vi "PMOD Example(FPGA).vi"() -> ()   [LabVIEW 2013]
uses:
  <vilib>/rvi/DataTransferAndStorage/Container/XNode/niFpgaContainer.xnode
  <vilib>/rvi/interface/RandomDataEmulation/nirviRandomDataFpgaReadWriteTemplate.vi
  <vilib>/Platform/TimedLoop/XDataNode/XDataNode.xnode
  <vilib>/Platform/TimedLoop/XDataNode/nitl_modes.ctl
  <vilib>/Platform/TimedLoop/XDataNode/XDNodeRunTimeDep.lvlib
  <vilib>/Platform/TimedLoop/XDataNode/wakeup.ctl
  <vilib>/Platform/TimedLoop/XDataNode/timing_clust.ctl
  DIO/SPI Digital IO Lines.ctl
  DIO/SPI DIO Enable Lines.ctl
  Controls/SPIExample.CurrentStateFPGA.ctl
  <userlib>/_NI SPI IP/FPGA/Controllers/Public/Spi Master Outputs.ctl
  <userlib>/_NI SPI IP/FPGA/Controllers/NI SPI IP (FPGA).lvlib
  <userlib>/_NI SPI IP/FPGA/Controllers/Public/Transfer Settings.ctl
panel:
  out "Raw ADC Data":u64
  out "read Iterations":i32
  in  "Data To ADC":u64=2147483648
  in  "Chip Select":u8
  in  "SPI PHY Settings":T1={"Divide Value"=20, "Transfer Length (bits)"=32, "CS Asserted Polarity"=FALSE, "Clock Polarity (CPOL)"=FALSE, "Clock Phase (CPHA)"=FALSE, "Lengthen MISO Setup"=FALSE, "Direction Change Bit"=0, "MOSI Starts as Output"=FALSE, "Tristatable MOSI"=FALSE} {"Direction Change Bit" max=64 step=1; "Transfer Length (bits)" min=1 max=64 step=1}
  out "spi output":T2
  in  "Chan Offset Array":sgl[](array[numeric])=[0.0, 0.0, 0.0, 0.0, 0.0, 0.0, 0.0, 0.0, 0.0, 0.0, 0.0, 0.0, 0.0, 0.0, 0.0, 0.0, 0.0, 0.0, 0.0, 0.0, 0.0, 0.0, 0.0, 0.0, 0.0, 0.0, 0.0, 0.0, 0.0, 0.0, 0.0, 0.0, 0.0, 0.0, 0.0, 0.0, 0.0, 0.0, 0.0, 0.0]
  out "SGL Data":sgl
  out "State":T3
  out "Iterations":i32
  in  "Debug":bool=TRUE
  out "Chan Count":bool
  out "oclk mult":u32
  in  "data rate (S/s)":u32=10000
  out "oclk freq":u32
  out "oclk div":u32
  in  "Chan Scale Array":sgl[](array[numeric])=[1.0, 1.0, 1.0, 0.0, 0.0, 0.0, 0.0, 0.0, 0.0, 0.0, 0.0, 0.0, 0.0, 0.0, 0.0, 0.0, 0.0, 0.0, 0.0, 0.0, 0.0, 0.0, 0.0, 0.0, 0.0, 0.0, 0.0, 0.0, 0.0, 0.0, 0.0, 0.0, 0.0, 0.0, 0.0, 0.0, 0.0, 0.0, 0.0, 0.0]
  out "FPGA Error":errorcluster
  out "Finished":bool
  in  "stop":bool
  out "Module Underflow":bool
  out "Acq Loop Ticks":u32
  out "DMA FIFO Full":bool
  out "First Read":bool
  in  "Number of Channels":i32=4
  in  "Acquisition Type":enum16{"Finite Samples", "Continuous Samples"}(ring)=enum."Continuous Samples"
  in  "Samps per Chan [Finite]":i32=5120
  # "OUTPUT"
  # "INPUT"
  # "ADC Data::Debug"
  # "Acquisition Parameters"
  # "SPI PHY Settings"
  # "Debug"
  # "Status"
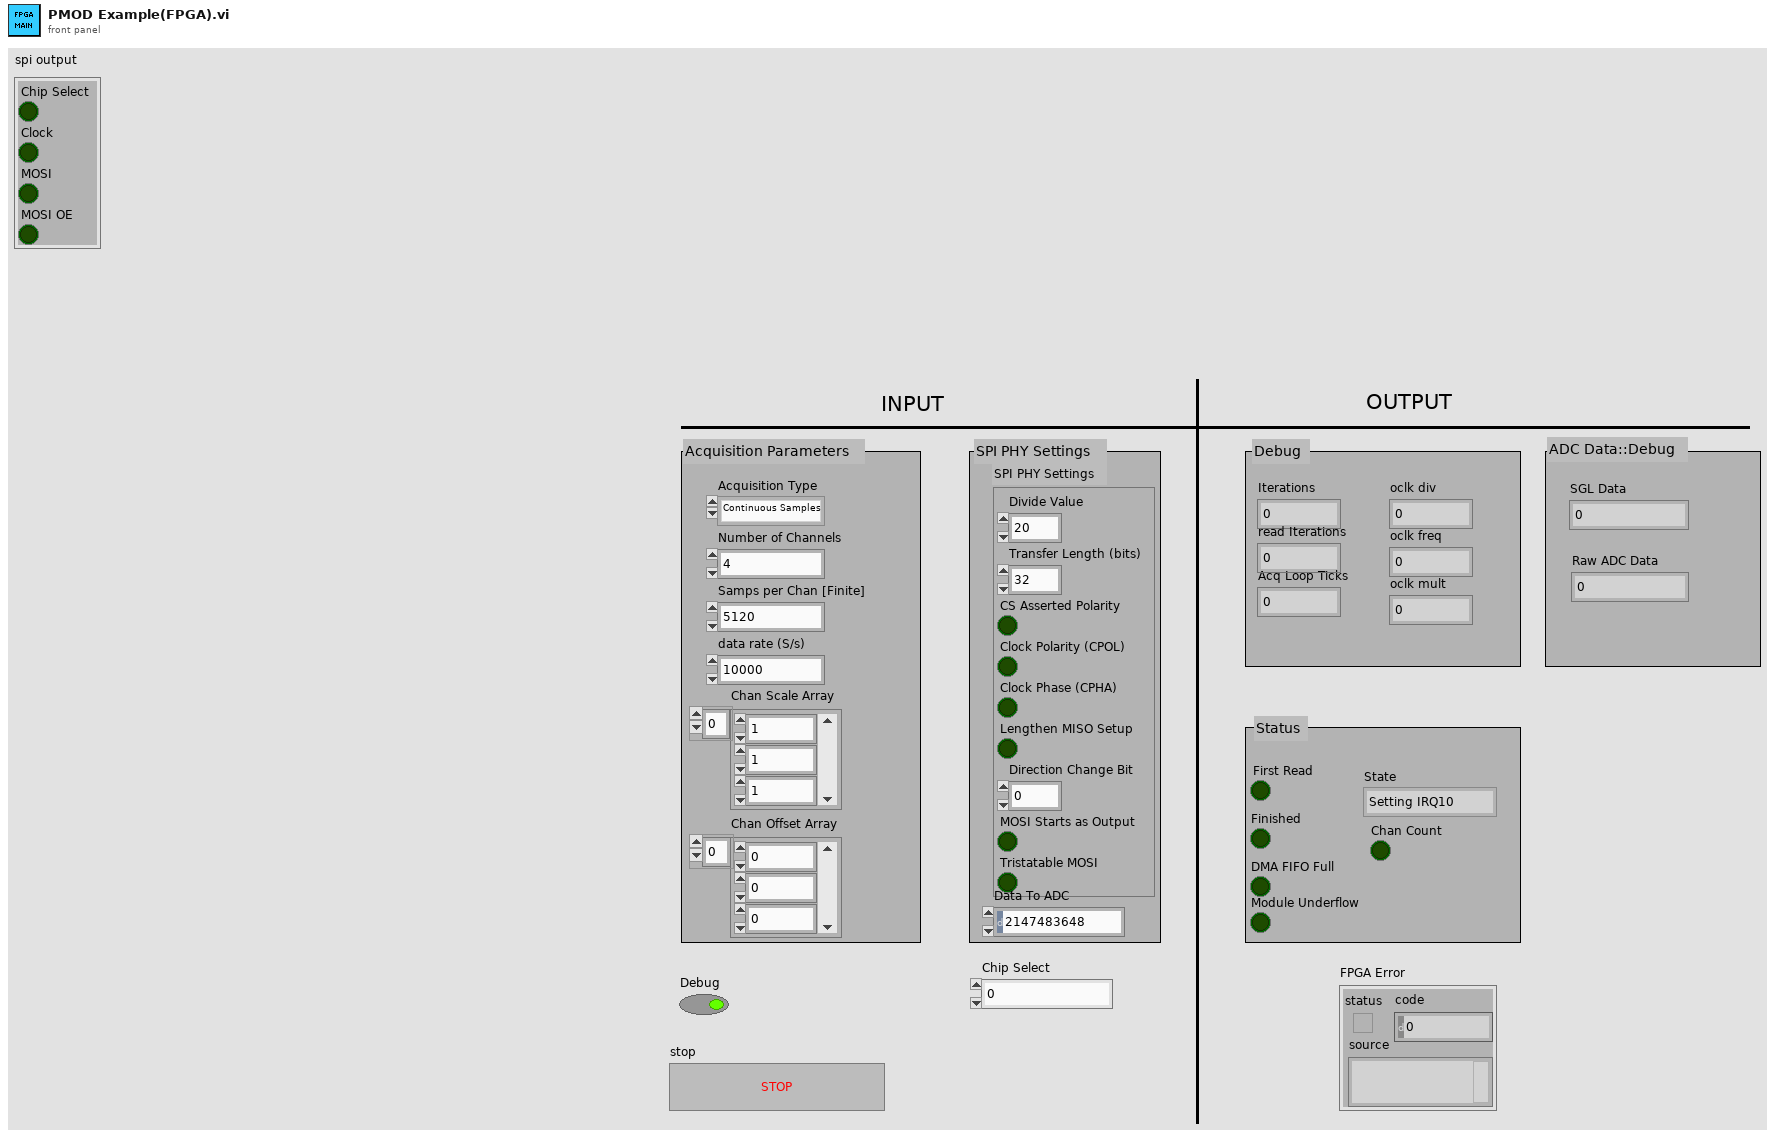
[diagram p1: front panel]
types:
  T1 = typedef "NI SPI IP (FPGA).lvlib/Transfer Settings.ctl" = cluster{"Divide Value":u8, "Transfer Length (bits)":u8, "CS Asserted Polarity":bool, "Clock Polarity (CPOL)":bool, "Clock Phase (CPHA)":bool, "Lengthen MISO Setup":bool, "Direction Change Bit":u8, "MOSI Starts as Output":bool, "Tristatable MOSI":bool}
  T2 = typedef "NI SPI IP (FPGA).lvlib/Spi Master Outputs.ctl" = cluster{"Chip Select":bool, "Clock":bool, "MOSI":bool, "MOSI OE":bool}
  T3 = typedef "SPIExample.CurrentStateFPGA.ctl" = enum16{"Setting IRQ10", "Config SPI", "Setting IRQ11", "Init Var", "IO Engine Running"}
  T4 = typedef "SPI DIO Enable Lines.ctl" = cluster{"SCLK_en":refnum<k21>, "MISO_en":refnum<k21>, "MOSI_en":refnum<k21>, "CS0_en":refnum<k21>, "CS1_en":refnum<k21>, "CS2_en":refnum<k21>, "CS3_en":refnum<k21>, "CS4_en":refnum<k21>, "CS5_en":refnum<k21>}
  T5 = typedef "SPI Digital IO Lines.ctl" = cluster{"SCLK":refnum<k21>, "MISO":refnum<k21>, "MOSI":refnum<k21>, "CS 0":refnum<k21>, "CS 1":refnum<k21>, "CS 2":refnum<k21>, "CS 3":refnum<k21>, "CS 4":refnum<k21>, "CS 5":refnum<k21>}
  T6 = typedef "XDNodeRunTimeDep.lvlib/timing_clust.ctl" = cluster{"Expected End [f-1]":u64, "Actual End [f-1]":u64, "Finished Late? [f-1]":bool, "Expected End [i-1]":u64, "Actual End [i-1]":u64, "Finished Late? [i-1]":bool, "Expected Start [i]":u64, "Actual Start [i]":u64, "Expected Start [f]":u64, "Actual Start [f]":u64, "Source Name":string, "Structure Name":string, "Period":i64, "Deadline":i64, "Offset":i64, "Start":i64, "Priority":i32, "Timeout":i32, "Mode":T7, "Wakeup Reason":T8, "Error":errorcluster, "Source Type":string, "Secondary Source Type":string, "Global End Time":u64, "Global Start Time":u64, "Frame Duration":u64, "Iteration Duration":u64, "Assigned CPU":i32, "I/O Scan Engine Mode":u32}
  T7 = typedef "XDNodeRunTimeDep.lvlib/nitl_modes.ctl" = enum32{"No Change", "Process missed periods, maintain original phase", "Discard missed periods, maintain original phase", "Process missed periods, ignore original phase", "Discard missed periods, ignore original phase"}
  T8 = typedef "XDNodeRunTimeDep.lvlib/wakeup.ctl" = enum32{"Normal", "Aborted", "Asynchronous wakeup", "Timing source error", "Timed loop error", "Timeout"}
  T9 = typedef "Internal Data (SPI API).ctl" = cluster{"DLU To SPI Engine Data FIFO":refnum<k21>, "SPI Engine to DLU Data FIFO":refnum<k21>, "Data to SPI Engine (Cache) Register":refnum<k21>, "SPI PHY Settings to SPI Engine (Cahche) Register":refnum<k21>}
  T10 = typedef "NI SPI IP (FPGA).lvlib/Spi Master Inputs.ctl" = cluster{"MISO":bool}
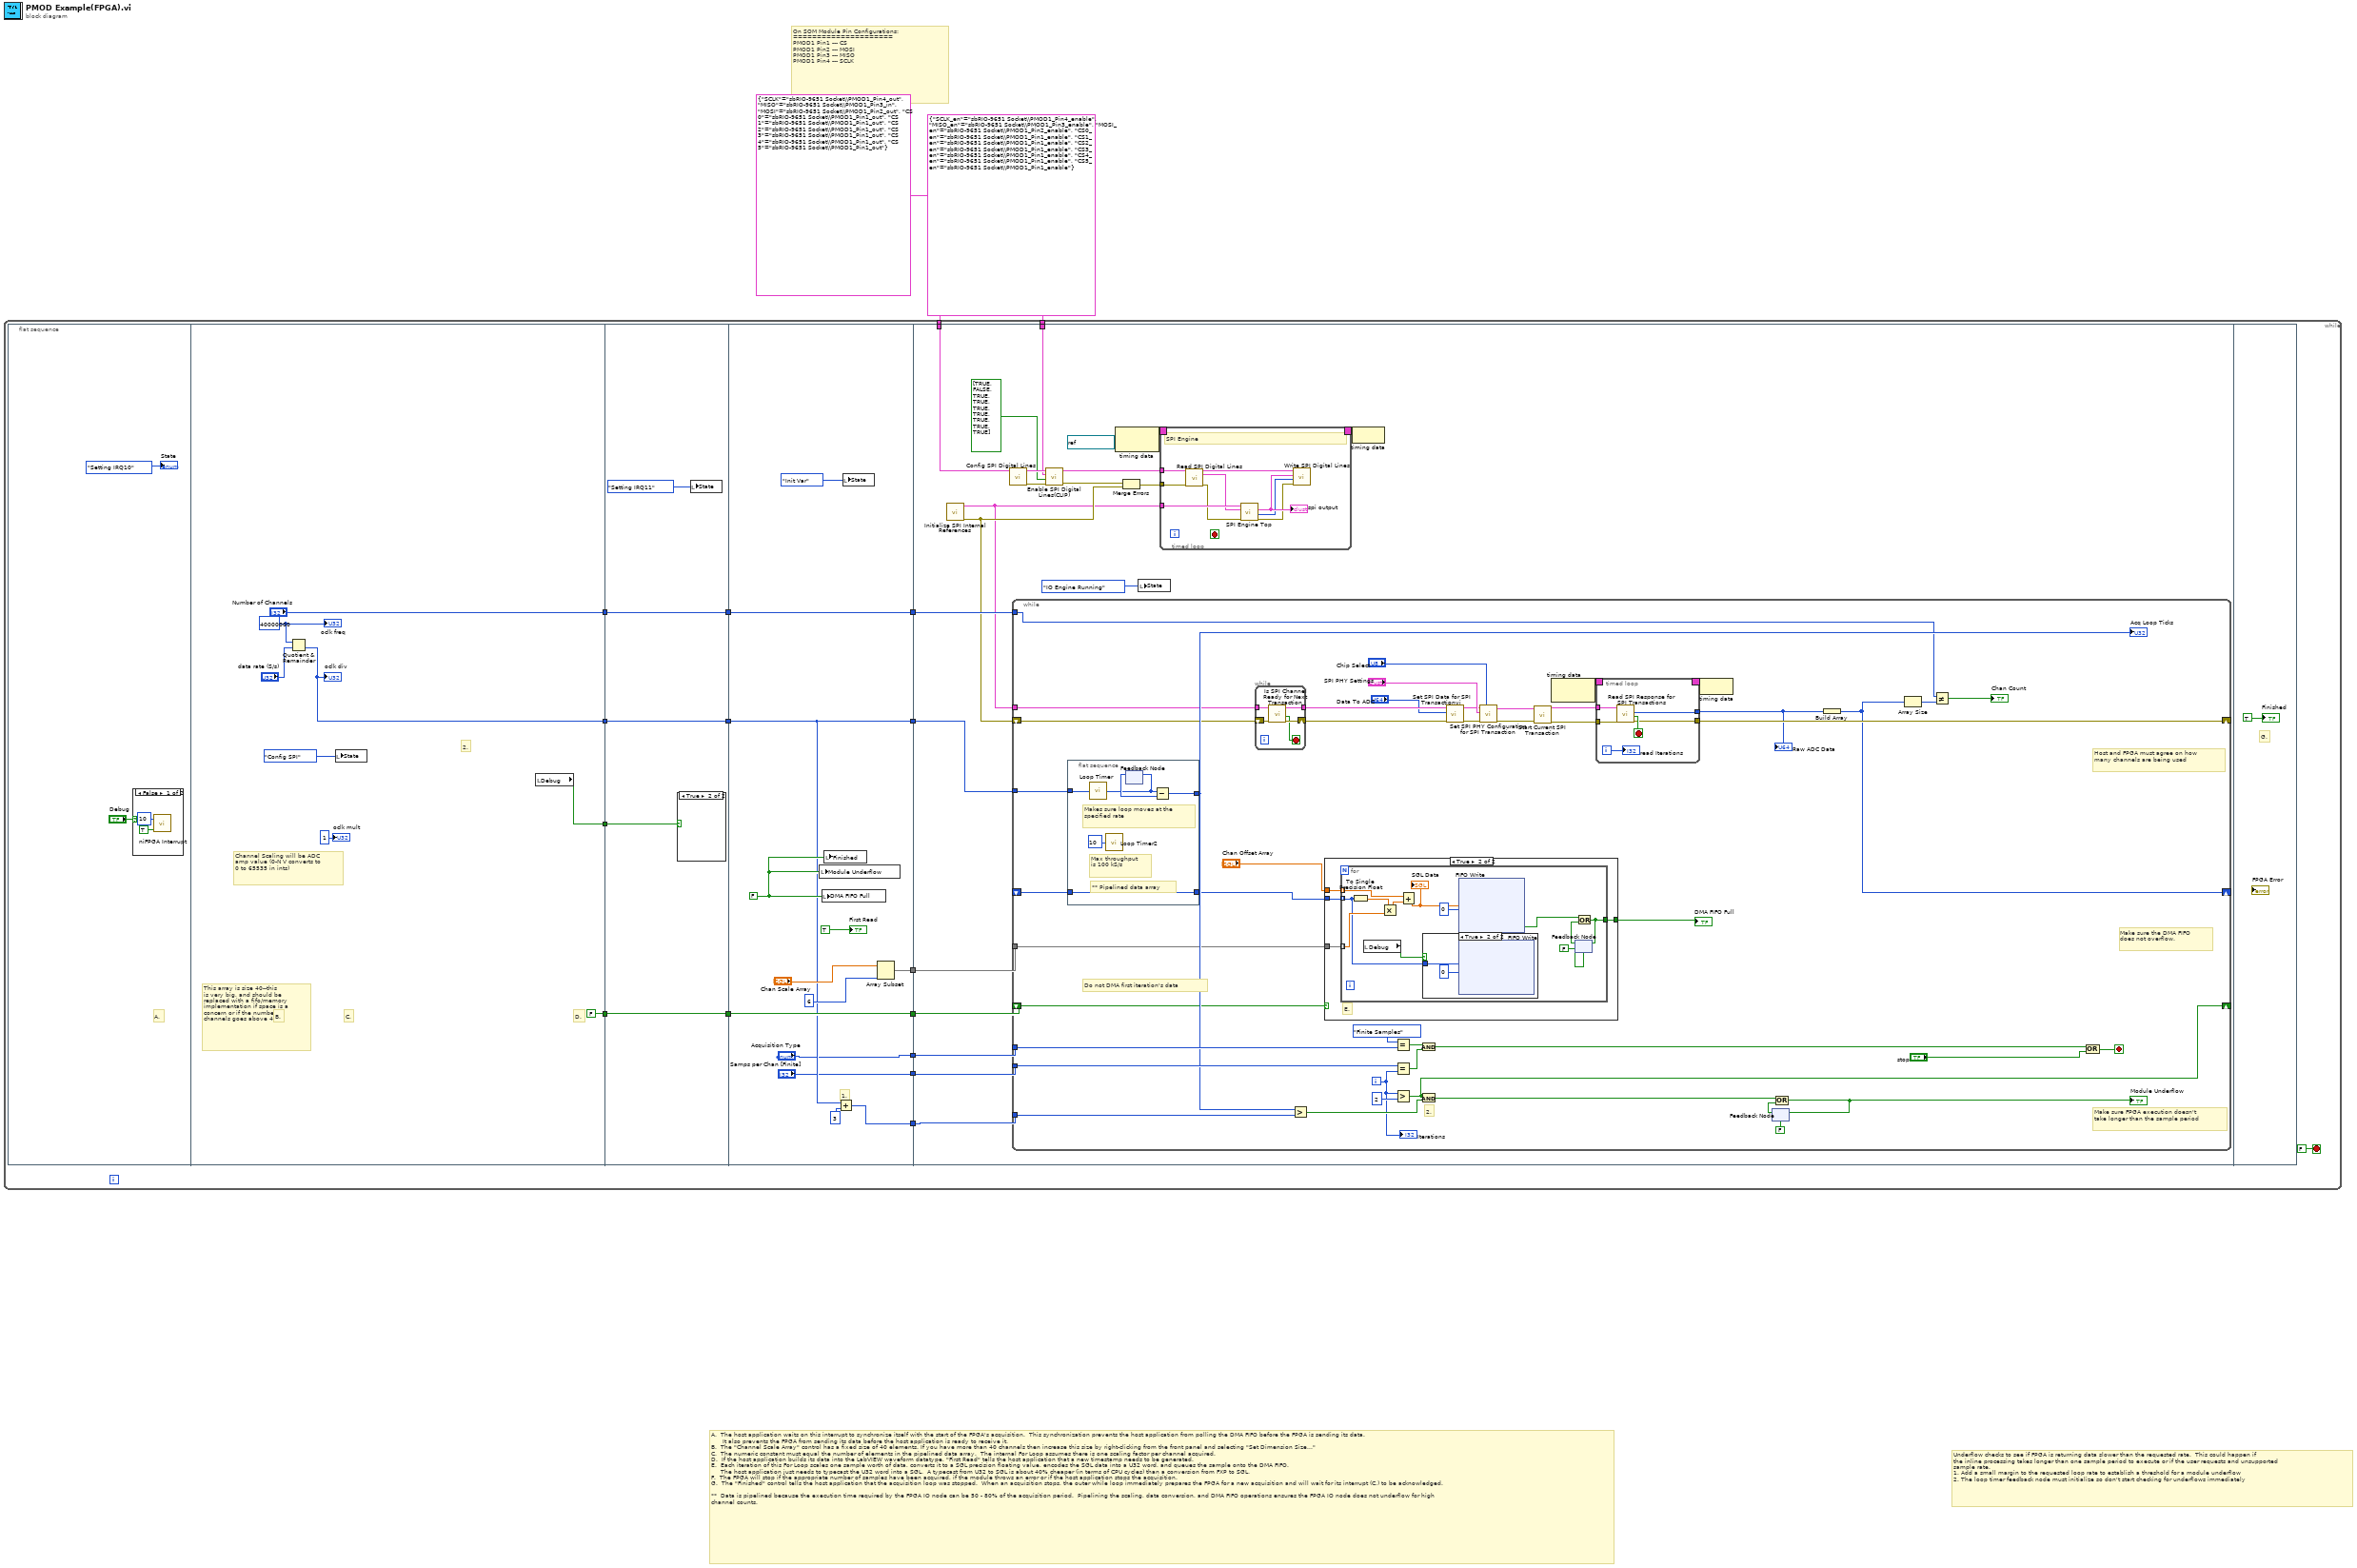
[diagram p0: block diagram]
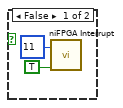
[diagram p3: hidden frame]
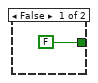
[diagram p4: hidden frame]
diagram:
  # "On SOM Module Pin Configurations:\n=====================\nPMOD1 Pin1 --- CS\nPMOD1 Pin2 --- MOSI\nPMOD1 Pin3 --- MISO\nPMOD1 Pin4 --- SCLK"
  # "Underflow checks to see if FPGA is returning data slower than the requested rate.  This could happen if\nthe inline processing takes longer than one sample period to execute or if the user requests and unsupported\nsample rate.\n1. Add a small margin to the requested loop rate to establish a threshold for a module underflow \n2. The loop timer feedback node must initialize so don't start checking for underflows immediately"
  # "A.  The host application waits on this interrupt to synchronize itself with the start of the FPGA's acquisition.  This synchronization prevents the host application from polling the DMA FIFO before the FPGA is sending its data.\n      It also prevents the FPGA from sending its data before the host application is ready to receive it.\nB.  The \"Channel Scale Array\" control has a fixed size of 40 elements. If you have more than 40 channels then increase this size by right-clicking from the front panel and selecting \"Set Dimension Size...\"\nC.  The numeric constant must equal the number of elements in the pipelined data array.  The internal For Loop assumes there is one scaling factor per channel acquired.\nD.  If the host application builds its data into the LabVIEW waveform datatype, \"First Read\" tells the host application that a new timestamp needs to be generated.\nE.  Each iteration of this For Loop scales one sample worth of data, converts it to a SGL precision floating value, encodes the SGL data into a U32 word, and queues the sample onto the DMA FIFO.  \n     The host application just needs to typecast the U32 word into a SGL.  A typecast from U32 to SGL is about 40% cheaper (in terms of CPU cycles) than a conversion from FXP to SGL.\nF.  The FPGA will stop if the appropriate number of samples have been acquired, if the module throws an error or if the host application stops the acquisition.  \nG.  The \"Finished\" control tells the host application that the acquisition loop was stopped.  When an acquisition stops, the outer while loop immediately prepares the FPGA for a new acquisition and will wait for its interrupt (C.) to be acknowledged. \n\n**  Data is pipelined because the execution time required by the FPGA IO node can be 50 - 80% of the acquisition period.  Pipelining the scaling, data conversion, and DMA FIFO operations ensures the FPGA IO node does not underflow for high\nchannel counts."
  n1 = while {
    tunnel: T5 {"SCLK"="sbRIO-9651 Socket\\PMOD1_Pin4_out", "MISO"="sbRIO-9651 Socket\\PMOD1_Pin3_in", "MOSI"="sbRIO-9651 Socket\\PMOD1_Pin2_out", "CS 0"="sbRIO-9651 Socket\\PMOD1_Pin1_out", "CS 1"="sbRIO-9651 Socket\\PMOD1_Pin1_out", "CS 2"="sbRIO-9651 Socket\\PMOD1_Pin1_out", "CS 3"="sbRIO-9651 Socket\\PMOD1_Pin1_out", "CS 4"="sbRIO-9651 Socket\\PMOD1_Pin1_out", "CS 5"="sbRIO-9651 Socket\\PMOD1_Pin1_out"} ("Chip Select DIO Lines") -> [w4]
    tunnel: T4 {"SCLK_en"="sbRIO-9651 Socket\\PMOD1_Pin4_enable", "MISO_en"="sbRIO-9651 Socket\\PMOD1_Pin3_enable", "MOSI_en"="sbRIO-9651 Socket\\PMOD1_Pin2_enable", "CS0_en"="sbRIO-9651 Socket\\PMOD1_Pin1_enable", "CS1_en"="sbRIO-9651 Socket\\PMOD1_Pin1_enable", "CS2_en"="sbRIO-9651 Socket\\PMOD1_Pin1_enable", "CS3_en"="sbRIO-9651 Socket\\PMOD1_Pin1_enable", "CS4_en"="sbRIO-9651 Socket\\PMOD1_Pin1_enable", "CS5_en"="sbRIO-9651 Socket\\PMOD1_Pin1_enable"} ("Enable Lines") -> [w3]
    stop <- FALSE stop-if-true
    n2 = flat-sequence {
      tunnel: ["Number of Channels"] -> w18
      tunnel: [FALSE] -> w17
      tunnel: [w27] -> w16
      tunnel: [w25] -> w5
      tunnel: w18 -> [w36]
      tunnel: [w36] -> w15
      tunnel: w17 -> [w35]
      tunnel: [w35] -> w9
      tunnel: w16 -> [w34]
      tunnel: [w34] -> w7
      tunnel: w5 -> [w33]
      tunnel: w15 -> [w51]
      tunnel: [w51] -> w14
      tunnel: [w47] -> w13
      tunnel: ["Acquisition Type"] -> w12
      tunnel: ["Samps per Chan [Finite]"] -> w11
      tunnel: [w43] -> w10
      tunnel: w9 -> [w50]
      tunnel: [w50] -> w8
      tunnel: w7 -> [w42]
      tunnel: [w42] -> w6
      tunnel: w14 -> [w72]
      tunnel: w13 -> [w70]
      tunnel: w12 -> [w69]
      tunnel: w11 -> [w68]
      tunnel: w10 -> [w67]
      tunnel: w8 -> [w66]
      tunnel: w6 -> [w71]
      tunnel: w4 -> [w53]
      tunnel: w3 -> [w52]
      frame #0 {
        # "A."
        n3 = case shown="False" "Debug" {
          frame False {
            n4 = call <vilib>:"niFPGA Interrupt.vi"("Wait Until Cleared (F)"=TRUE ("Wait Until Cleared"), "IRQ Number (0)"=u8 10 ("IRQ Number")) -> ()  [unwired: 1 in]
          }
          frame True {
          }
        }
        "State" <- SPIExample.CurrentStateFPGA."Setting IRQ10" ("State")
      }
      frame #1 {
        w28 = u32 40000000 ("oclk freq")
        # "2."
        # "This array is size 40--this\nis very big, and should be\nreplaced with a fifo/memory\nimplementation if space is a\nconcern or if the number of \nchannels goes above 40"
        # "Channel Scaling will be ADC\namp value (0-N V converts to\n0 to 65535 in ints)"
        # "D."
        # "C."
        # "B."
        n5 = Quotient & Remainder(x=w28, y="data rate (S/s)") -> (floor(x/y)=w27:u32)  [unwired: 1 out]
        "oclk div" <- w27
        n6 = local write "State"(SPIExample.CurrentStateFPGA."Config SPI" ("State")) -> ()
        n7 = local read "Debug"() -> (w25:bool)
        "oclk freq" <- w28
        "oclk mult" <- u32 1 ("oclk mult")
      }
      frame #2 {
        n8 = case shown="True" w33 {
          frame False {
            n9 = call <vilib>:"niFPGA Interrupt.vi"("Wait Until Cleared (F)"=TRUE ("Wait Until Cleared"), "IRQ Number (0)"=u8 11 ("IRQ Number")) -> ()  [unwired: 1 in]
          }
          frame True {
          }
        }
        n10 = local write "State"(SPIExample.CurrentStateFPGA."Setting IRQ11" ("State")) -> ()
      }
      frame #3 {
        w49 = FALSE ("Module Underflow")
        # "1."
        n11 = local write "Module Underflow"(w49) -> ()
        n12 = local write "DMA FIFO Full"(w49) -> ()
        n13 = local write "Finished"(w49) -> ()
        n14 = Add(x=w42, y=u32 3) -> (x+y=w43:u32)
        n15 = local write "State"(SPIExample.CurrentStateFPGA."Init Var" ("State")) -> ()
        n16 = Array Subset(array="Chan Scale Array", length=6) -> (w47:sgl[])  [unwired: 1 in]
        "First Read" <- TRUE ("First Read")
      }
      frame #4 {
        n17 = call "Initialize SPI Internal References.vi"() -> ("error out"=w64:errorcluster, "SPI API References"=w63:T9)  [unwired: 10 in]
        n18 = call "Config SPI Digital Lines.vi"("SPI DIO Lines"=w53) -> ("error out"=w55:errorcluster, "Chip Select DIO Lines"=w56:T5)  [unwired: 9 in]
        n19 = while {
          tunnel: w69 -> [w129]
          tunnel: w68 -> [w128]
          shift-right: [w99] -> _
          shift-left: _ -> [w122]
          tunnel: w72 -> [w107]
          tunnel: w71 -> [w127]
          tunnel: w67 -> [w124]
          tunnel: w70 -> [w112]
          shift-right: [w111] -> _
          shift-left: w66 -> [w121]
          shift-right: [w101] -> _
          shift-left: w64 -> [w102]
          tunnel: w63 -> [w103]
          i -> [w120]
          stop <- w131 stop-if-true
          # "2."
          # "Do not DMA first iteration's data"
          # "Host and FPGA must agree on how \nmany channels are being used"
          # "Make sure the DMA FIFO\ndoes not overflow."
          # "Make sure FPGA execution doesn't\ntake longer than the sample period"
          n20 = flat-sequence {
            tunnel: w127 -> [w173]
            tunnel: [w170] -> w123
            tunnel: [w169] -> w110
            tunnel: w122 -> [w169]
            frame #0 {
              # "Max throughput\nis 100 kS/s"
              # "Makes sure loop moves at the\nspecified rate"
              # "** Pipelined data array"
              n21 = call "Loop Timer"("Count(Ticks)"=w173) -> ("Tick Count(Ticks)"=w171:u32)
              n22 = call "Loop Timer2"("Count(uSec)"=u8 10 ("Count(Ticks)")) -> ()  [unwired: 1 out]
              n23 = feedback-in #1(w171) -> ()
              n24 = feedback #1() -> (w172:u32)  [unwired: 1 out]
              n25 = Subtract(x=w171, y=w172) -> (x-y=w170:u32)
            }
          }
          n26 = while {
            shift-right: [w138] -> w105
            shift-left: w102 -> [w135]
            tunnel: w103 -> [w136]
            tunnel: [w137] -> w104
            stop <- w134 stop-if-true
            n27 = call "Is SPI Channel Ready for Next Transaction.vi"("error in"=w135, "Private Data In"=w136) -> ("error out"=w138:errorcluster, "SPI Channel Ready"=w134:bool, "Private Data Out"=w137:T9)  [unwired: 6 in, 1 out]
          }
          n28 = Greater?(x=w123, y=w124) -> (0:w126:bool)
          n29 = case shown="True" w121 {
            tunnel: [FALSE w153] -> w130
            tunnel: w110 -> [_ w152]
            tunnel: w112 -> [_ w151]
            tunnel: "Chan Offset Array" -> [_ w150]
            frame False {
            }
            frame True {
              # "E."
              n30 = for {
                tunnel: [w162] -> w153
                tunnel: w152 -> [w154] mode=indexing
                tunnel: w151 -> [w160] mode=indexing
                tunnel: w150 -> [w155] mode=indexing
                n31 = To Single Precision Float(number=w154) -> (single precision float=w158:sgl)
                n32 = local read "Debug"() -> (w157:bool)
                n33 = Multiply(x=w158, y=w160) -> (x*y=w159:sgl)
                n34 = Add(x=w155, y=w159) -> (x+y=w156:sgl)
                "SGL Data" <- w156
                n35 = case shown="True" w157 {
                  tunnel: w154 -> [_ w166]
                  frame False {
                  }
                  frame True {
                    n36 = xnode ("FIFO Write")("Element"=w166, "Timeout"=0) -> ()  [unwired: 1 in, 2 out]
                  }
                }
                n37 = xnode ("FIFO Write")("Element"=w156, "Timeout"=0) -> ("Timed Out?"=w165:bool)  [unwired: 1 in, 1 out]
                n38 = feedback #2(FALSE) -> (w163:bool)
                n39 = Or(x=w165, y=w163) -> (x .or. y?=w162:bool)
                n40 = feedback-in #2(w162) -> ()
              }
            }
          }
          "DMA FIFO Full" <- w130
          n41 = Equal?(x=enum16{"Finite Samples", "Continuous Samples"}."Finite Samples" ("y"), y=w129) -> (x = y?=w115:bool)
          n42 = Equal?(x=w128, y=w120) -> (x = y?=w114:bool)
          n43 = Greater?(x=w120, y=2) -> (0:w111:bool)
          n44 = And(x=w115, y=w114) -> (x .and. y?=w113:bool)
          n45 = And(x=w111, y=w126) -> (x .and. y?=w117:bool)
          n46 = call "Set SPI Data for SPI Transactionvi.vi"("error in"=w105, "Data In"="Data To ADC", "Private Data In"=w104) -> ("error out"=w93:errorcluster, "Private Data Out"=w94:T9)  [unwired: 7 in]
          n47 = call "Set SPI PHY Configuration for SPI Transaction.vi"("Chip Select"="Chip Select", "error in"=w93, "SPI PHY Settings"="SPI PHY Settings", "Private Data In"=w94) -> ("error out"=w90:errorcluster, "Private Data Out"=w91:T9)  [unwired: 6 in]
          n48 = call "Start Current SPI Transaction.vi"("error in"=w90, "Private Data In"=w91) -> ("error out"=w95:errorcluster, "Private Data Out"=w89:T9)  [unwired: 7 in, 1 out]
          n49 = node-c288() -> (w98:T6)  [unwired: 1 in]
          n50 = timed-loop {
            timing: w98 -> [_]
            timing-out: [_] -> w97
            tunnel: w95 -> [w144]
            tunnel: w89 -> [w143]
            tunnel: [w141] -> w100
            tunnel: [w140] -> w101
            i -> [w139]
            stop <- w142 stop-if-true
            n51 = call "Read SPI Response for SPI Transactions.vi"("error in"=w144, "Private Data In"=w143) -> ("error out"=w140:errorcluster, "Read Data Valid?"=w142:bool, "Read Data"=w141:u64)  [unwired: 6 in, 1 out]
            "read Iterations" <- w139
          }
          "Raw ADC Data" <- w100
          n52 = node-c288(w97) -> ()
          n53 = feedback #3(FALSE) -> (w119:bool)
          n54 = Or(x=w117, y=w119) -> (x .or. y?=w116:bool)
          "Module Underflow" <- w116
          n55 = feedback-in #3(w116) -> ()
          n56 = Build Array(w100) -> (w99:u64[])
          n57 = Array Size(array=w99) -> (size(s)=w109:i32)
          n58 = Not Equal?(x=w107, y=w109) -> (x != y?=→"Chan Count":bool)
          n59 = Compound Arithmetic op=OR(w113, "stop") -> (w131:bool)
          "Acq Loop Ticks" <- w123
          "Iterations" <- w120
        }
        n60 = call "Enable SPI Digital Lines(CLIP).vi"("error in"=w55, "Enable"=bool[] [TRUE, FALSE, TRUE, TRUE, TRUE, TRUE, TRUE, TRUE, TRUE], "Enable Lines"=w52, "SPI DIO Lines"=w56) -> ("error out"=w57:errorcluster, "Chip Select DIO Lines"=w58:T5)  [unwired: 6 in]
        n61 = node-c288(refnum<k21> "120MHz" ("Source Name")) -> (w62:T6)
        n62 = Merge Errors(w57, w64) -> (w60:errorcluster)
        n63 = local write "State"(SPIExample.CurrentStateFPGA."IO Engine Running" ("State")) -> ()
        n64 = timed-loop {
          tunnel: w63 -> [w78]
          tunnel: w60 -> [w76]
          tunnel: w58 -> [w80]
          timing: w62 -> [_]
          timing-out: [_] -> w61
          stop <- _ stop-if-true
          # "SPI Engine"
          n65 = call "Read SPI Digital Lines.vi"("Chip Select DIO Lines"=w80, "error in"=w76) -> ("Chip Select DIO Lines Out"=w81:T5, "SPI Read Data"=w77:T10, "error out"=w75:errorcluster)  [unwired: 11 in]
          n66 = call "SPI Engine Top.vi"("error in"=w75, "SPI Read Data"=w77, "SPI API References"=w78) -> ("error out"=w74:errorcluster, "Chip Select ID"=w73:u8, "SPI DIO Output"=w79:T2)  [unwired: 3 in, 3 out]
          "spi output" <- w79
          n67 = call "Write SPI Digital Lines.vi"("error in"=w74, "CS Index"=w73, "spi output"=w79, "Chip Select DIO Lines"=w81) -> ()  [unwired: 6 in, 2 out]
        }
        n68 = node-c288(w61) -> ()
      }
      frame #5 {
        # "G."
        "Finished" <- TRUE ("Finished")
      }
    }
  }
